vi "Copy LogFile to Location.vi"(5 "Local Save Path in":path, 7 "Log File Path in":path, 8 "error in":errorcluster, 11 "Target Information in":T1) -> (0 "error out":errorcluster, 1 "File Succesfuly copied":bool, 2 "Local Save Path out":path, 3 "Target Information out":T1)   [LabVIEW 2026, in "Telemetry System Tests.lvclass"]
uses:
  Telemetry System Tests.lvclass
  <vilib>/WebDAVClient/NI_WebDAV.lvlib
  <vilib>/WebDAVClient/Advanced/Get File.vi
  <vilib>/NI/VeriStand Custom Device Testing Tools/VeriStandTestUtilities/ChassisInformation.ctl
  <vilib>/NI/VeriStand Custom Device Testing Tools/VeriStandTestUtilities/VeriStandTestUtilities.lvlib
  <vilib>/NI/VeriStand Custom Device Testing Tools/VeriStandTestUtilities/TargetInformation.ctl
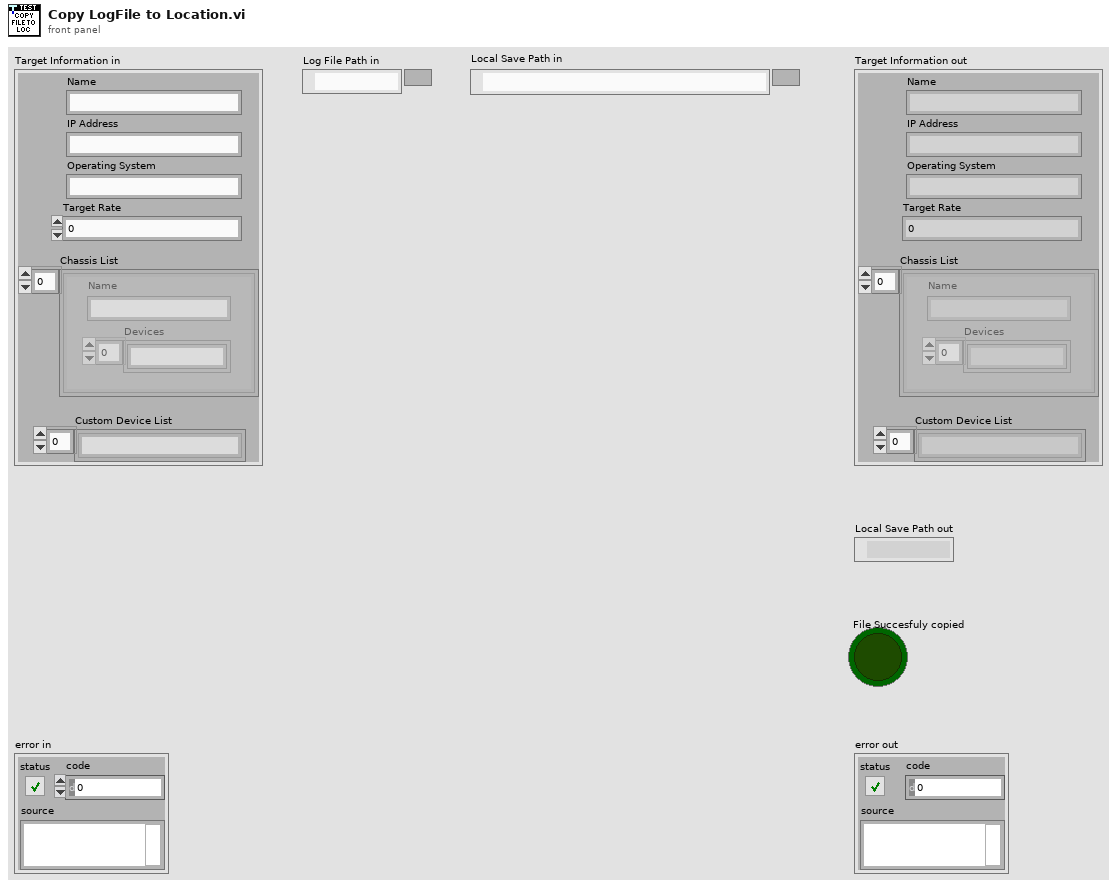
[diagram p1: front panel]
types:
  T1 = typedef "VeriStandTestUtilities.lvlib/TargetInformation.ctl" = cluster{"Name":string, "IP Address":string, "Operating System":string, "Target Rate":dbl, "Chassis List":T2[], "Custom Device List":string[]}
  T2 = typedef "VeriStandTestUtilities.lvlib/ChassisInformation.ctl" = cluster{"Name":string, "Devices":string[]}
  T3 = typedef "NI_WebDAV.lvlib/SessionHandle.ctl" = refnum<k1>
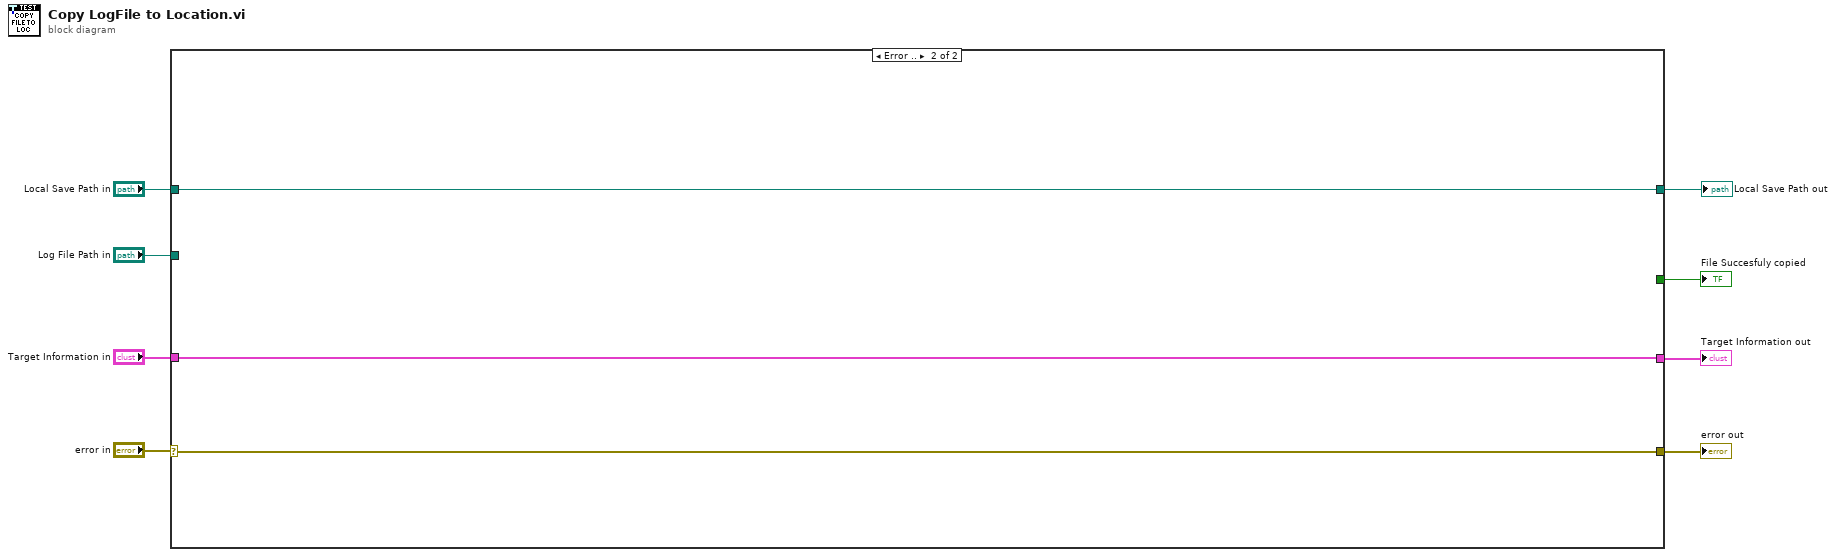
[diagram p0: block diagram]
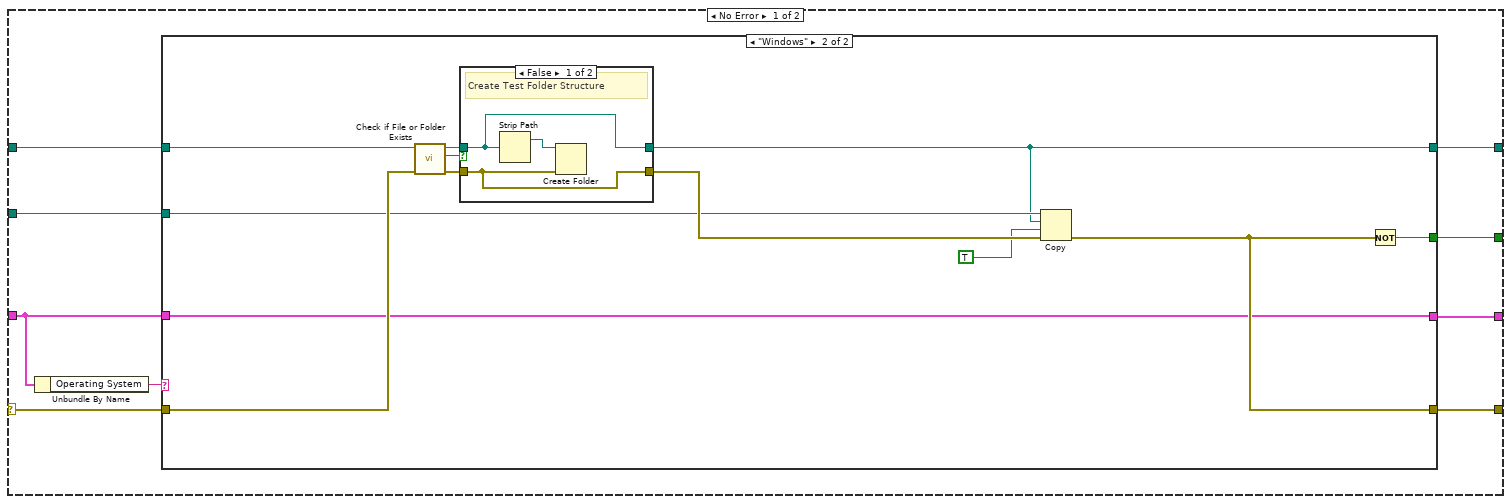
[diagram p2: hidden frame]
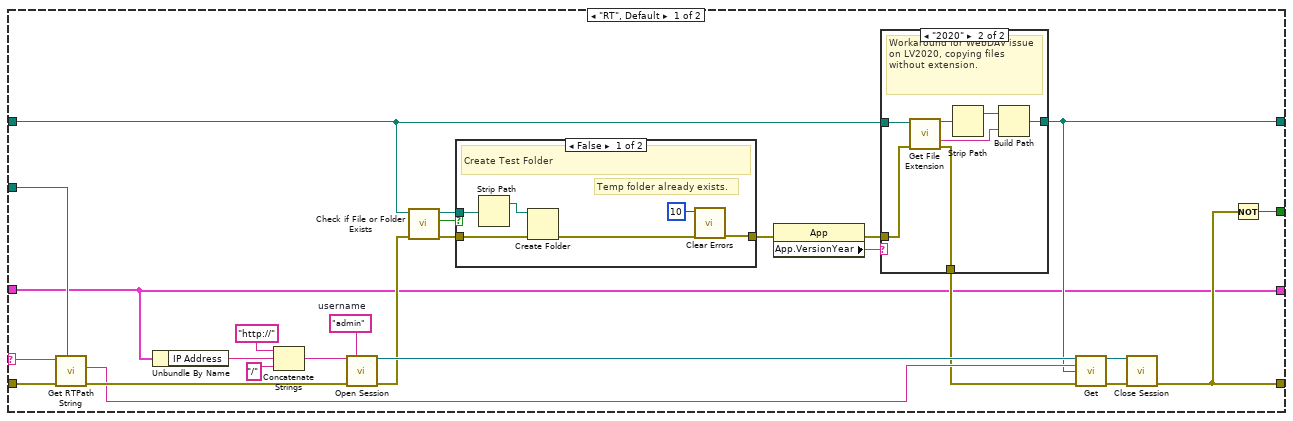
[diagram p3: hidden frame]
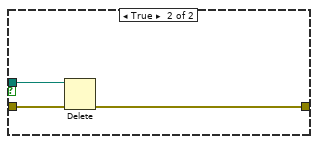
[diagram p5: hidden frame]
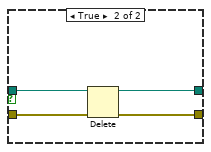
[diagram p6: hidden frame]
diagram:
  n1 = case shown="Error .." "error in" {
    selector: "error in" -> [w15 w83]
    tunnel: "Log File Path in" -> [w17 _]
    tunnel: "Target Information in" -> [w11 w82]
    tunnel: [w16 w83] -> w6
    tunnel: "Local Save Path in" -> [w14 w81]
    tunnel: [w13 _] -> w4
    tunnel: [w10 w81] -> w2
    tunnel: [w9 w82] -> w1
    frame No Error {
      n2 = Unbundle By Name(w11) -> ("Operating System"=w12:string)
      n3 = case shown="\"Windows\"" w12 {
        selector: w12 -> [w43 _]
        tunnel: [w29 w66] -> w16
        tunnel: w15 -> [w42 w73]
        tunnel: w17 -> [w26 w64]
        tunnel: w14 -> [w25 w69]
        tunnel: [w28 w65] -> w13
        tunnel: w11 -> [w18 w62]
        tunnel: [w23 w63] -> w10
        tunnel: [w18 w62] -> w9
        frame "RT", Default {
          w22 = "admin"  # username
          n4 = call "Get RTPath String.vi"("SysDef Log File Path"=w26, "error in (no error)"=w42, "Target OS in"=w43) -> ("error out"=w41:errorcluster, "RT File Path"=w30:string)  [unwired: 5 in, 2 out]
          n5 = Unbundle By Name(w18) -> ("IP Address"=w27:string)
          n6 = Concatenate Strings("http://" ("string"), w27, "/" ("string")) -> (w38:string)
          n7 = call <vilib>:"Open Session.vi"("host uri prefix"=w38, "username"=w22, "error in (no error)"=w41) -> ("session handle out"=w37:T3, "error out"=w34:errorcluster)  [unwired: 11 in]
          n8 = call <vilib>:"Check if File or Folder Exists.vi"("error in (no error)"=w34, "path"=w25) -> ("error out"=w31:errorcluster, "file or folder exists?"=w33:bool, "dup path"=w32:path)  [unwired: 7 in]
          n9 = case shown="False" w33 {
            tunnel: w32 -> [w58 w61]
            tunnel: w31 -> [w57 w60]
            tunnel: [w55 w59] -> w20
            frame False {
              # "Temp folder already exists."
              # "Create Test Folder"
              n10 = Strip Path(path=w58) -> (stripped path=w56:path)  [unwired: 1 out]
              n11 = Create Folder(path (use dialog)=w56, error in=w57) -> (error out=w54:errorcluster)  [unwired: 1 in, 2 out]
              n12 = call <vilib>:"Clear Errors.vi"("error in (no error)"=w54, "specific error code to clear (0: all)"=10) -> ("error out"=w55:errorcluster)  [unwired: 4 in, 1 out]
            }
            frame True {
              n13 = Delete(path (use dialog)=w61, error in=w60) -> (error out=w59:errorcluster)  [unwired: 3 in, 2 out]
            }
          }
          n14 = property class="App"(error in=w20) -> (error out=w21:errorcluster, "App.VersionYear"=w19:string)  [unwired: 1 in, 1 out]
          n15 = case shown="\"2020\"" w19 {
            tunnel: w25 -> [w45 w52]
            tunnel: w21 -> [w44 w51]
            tunnel: [w44 w50] -> w24
            tunnel: [w45 w49] -> w23
            frame Default {
            }
            frame "2020" {
              # "Workaround for WebDAV issue on LV2020, copying files without extension."
              n16 = call <vilib>:"Get File Extension.vi"("error in (no error)"=w51, "file"=w52) -> ("error out"=w50:errorcluster, "filename without extension"=w46:string, "dup file"=w48:path)  [unwired: 5 in, 2 out]
              n17 = Strip Path(path=w48) -> (stripped path=w47:path)  [unwired: 1 out]
              n18 = Build Path(base path=w47, name or relative path=w46) -> (appended path=w49:path)
            }
          }
          n19 = call-poly <vilib>:"Get.vi"("session handle"=w37, "relative uri"=w30, "local file path"=w23, "error in (no error)"=w24) -> ("session handle out"=w36:T3, "error out"=w35:errorcluster)  [unwired: 9 in, 1 out]
          n20 = call <vilib>:"Close Session.vi"("session handle"=w36, "error in (no error)"=w35) -> ("error out"=w29:errorcluster)  [unwired: 13 in]
          n21 = Not(x=w29) -> (.not. x?=w28:bool)
        }
        frame "Windows" {
          n22 = call <vilib>:"Check if File or Folder Exists.vi"("error in (no error)"=w73, "path"=w69) -> ("error out"=w70:errorcluster, "file or folder exists?"=w72:bool, "dup path"=w71:path)  [unwired: 7 in]
          n23 = case shown="False" w72 {
            tunnel: w71 -> [w75 w80]
            tunnel: w70 -> [w74 w79]
            tunnel: [w74 w78] -> w68
            tunnel: [w75 w77] -> w63
            frame False {
              # "Create Test Folder Structure"
              n24 = Strip Path(path=w75) -> (stripped path=w76:path)  [unwired: 1 out]
              n25 = Create Folder(path (use dialog)=w76, error in=w74) -> ()  [unwired: 1 in, 3 out]
            }
            frame True {
              n26 = Delete(path (use dialog)=w80, error in=w79) -> (deleted path=w77:path, error out=w78:errorcluster)  [unwired: 3 in, 1 out]
            }
          }
          n27 = Copy(8:w68, 9:TRUE ("overwrite (F)"), 10:w63, 11:w64) -> (0:w66:errorcluster)  [unwired: 1 in, 2 out]
          n28 = Not(x=w66) -> (.not. x?=w65:bool)
        }
      }
    }
    frame Error {
    }
  }
  "error out" <- w6
  "File Succesfuly copied" <- w4
  "Local Save Path out" <- w2
  "Target Information out" <- w1
